vi "Start Process.vi"(8 "error in (no error)":errorcluster, 11 "Process Model in":refnum<class "Process Model.lvclass">) -> (0 "error out":errorcluster, 3 "Process Model out":refnum<class "Process Model.lvclass">)   [LabVIEW 2017, in "Car Wash.lvlib" / "Process Model.lvlib" / "Process Model.lvclass"]
uses:
  Process Model.lvclass
  <vilib>/ActorFramework/Actor/Actor.lvclass
  D:/Project/General VIs/Process/iProcess Model/iProcess Model/iProcess Model.lvclass
  C:/Program Files/National Instruments/LabVIEW 2017/vi.lib/gpm_packages/@cs/mva-core/Source/IModel/IModel/IModel.lvclass
  C:/Program Files/National Instruments/LabVIEW 2017/vi.lib/gpm_packages/@cs/mva-core/Source/IObserver/IObserver/IObserver.lvclass
  C:/Program Files/National Instruments/LabVIEW 2017/vi.lib/ActorFramework/Actor/Actor.lvclass
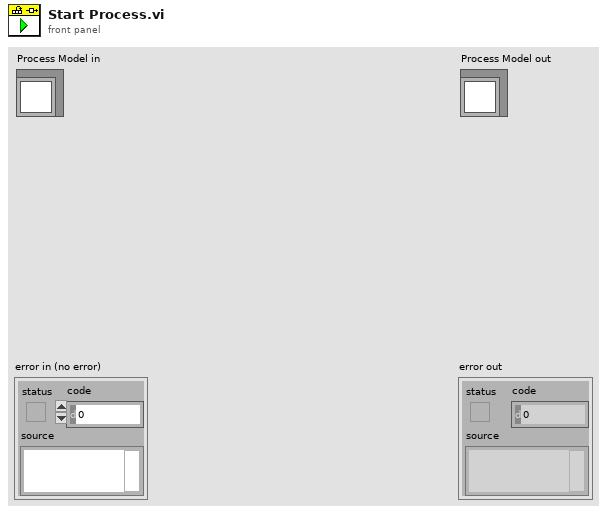
[diagram p1: front panel]
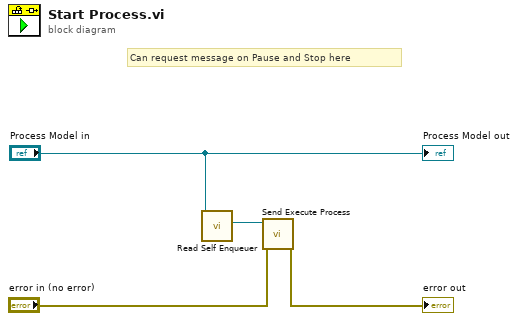
[diagram p0: block diagram]
diagram:
  # "Can request message on Pause and Stop here"
  n1 = call <vilib>:"Read Self Enqueuer.vi"("Actor"="Process Model in") -> ("Self Enqueuer"=w3:refnum<class "Message Enqueuer.lvclass">)  [unwired: 10 in]
  n2 = call "Send Execute Process.vi"("error in (no error)"="error in (no error)", "Message Enqueuer"=w3) -> ("error out"=→"error out":errorcluster)  [unwired: 8 in, 1 out]
  "Process Model out" <- "Process Model in"
